vi "Lab3.vi"() -> ()   [LabVIEW 2021]
panel:
  out "Error":dbl
  out "Estimation":dbl
  out "Exact":dbl
  in  "Iterations":dbl
  in  "X":dbl
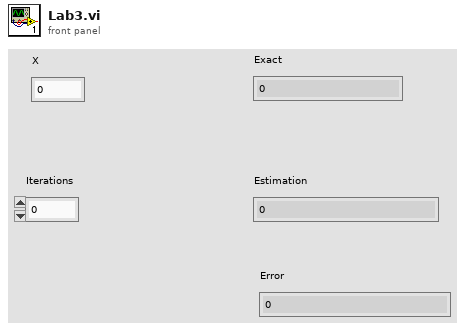
[diagram p1: front panel]
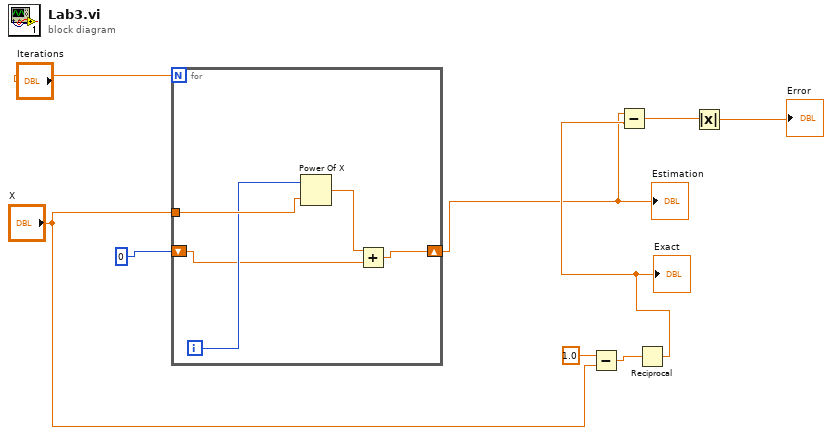
[diagram p0: block diagram]
diagram:
  n1 = for {
    N: "Iterations" -> [_]
    tunnel: "X" -> [w14]
    shift-right: [w10] -> w1
    shift-left: 0 -> [w12]
    i -> [w13]
    n2 = Power Of X(1:w14, 2:w13) -> (0:w11:dbl)
    n3 = Add(x=w11, y=w12) -> (x+y=w10:dbl)
  }
  "Estimation" <- w1
  n4 = Subtract(x=1.0, y="X") -> (x-y=w3:dbl)
  n5 = Reciprocal(x=w3) -> (1/x=w4:dbl)
  "Exact" <- w4
  n6 = Subtract(x=w1, y=w4) -> (x-y=w9:dbl)
  n7 = Absolute Value(x=w9) -> (abs(x)=→"Error":dbl)
